vi "MBwaitForSerialRegisters.vi"(10 "Decimal points (0)":u8[](array[numeric]), 11 "Serial port (0)":i32) -> (1 "CRC":u16, 2 "Process values":dbl[](array[numeric]) format="%.2f", 3 "String received from device":string)   [LabVIEW 2010]
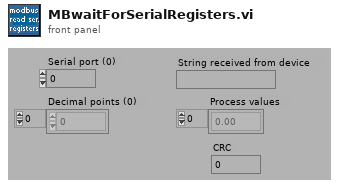
[diagram p1: front panel]
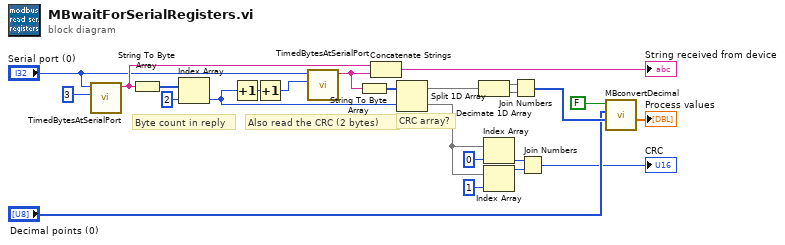
[diagram p0: block diagram]
diagram:
  # "Byte count in reply"
  # "Also read the CRC (2 bytes)"
  # "CRC array?"
  n1 = call "TimedBytesAtSerialPort.vi"("Byte count"=u32 3, "Serial port (0)"="Serial port (0)") -> ("String read"=w22:string)  [unwired: 1 in, 8 out]
  n2 = String To Byte Array(string=w22) -> (unsigned byte array=w14:u8[])
  n3 = Index Array(array=w14, index=2) -> (element=w19:u8)
  n4 = Increment(x=w19) -> (x+1=w17:u8)
  n5 = Increment(x=w17) -> (x+1=w18:u8)
  n6 = call "TimedBytesAtSerialPort.vi"("Byte count"=w18, "Serial port (0)"="Serial port (0)") -> ("String read"=w23:string)  [unwired: 1 in, 8 out]
  n7 = String To Byte Array(string=w23) -> (unsigned byte array=w20:u8[])
  n8 = Concatenate Strings(w22, w23) -> (→"String received from device":string)
  n9 = Split 1D Array(array=w20, index=w19) -> (first subarray=w21:u8[], second subarray=w6:u8[])
  n10 = Decimate 1D Array(w21) -> (w8:u8[], w9:u8[])
  n11 = Index Array(array=w6, index=0) -> (element=w3:u8)
  n12 = Index Array(array=w6, index=1) -> (element=w2:u8)
  n13 = Join Numbers(hi=w8, lo=w9) -> ((hi.lo)=w12:u16[])
  n14 = Join Numbers(hi=w3, lo=w2) -> ((hi.lo)=→"CRC":u16)
  n15 = call "MBconvertDecimal.vi"("Values"=w12, "Decimal points"="Decimal points (0)", "From (F) / to (T) decimal"=FALSE) -> ("New values"=→"Process values":dbl[])  [unwired: 8 out]
